vi "FGV RDB.vi"(9 "Raw data in":dbl[][](array[numeric]), 11 "Command":T1) -> (1 "Raw data out":dbl[][](array[numeric]), 3 "Size":i32)   [LabVIEW 2014]
uses:
  set-get-size.ctl
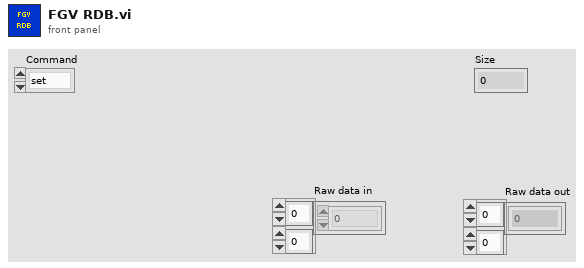
[diagram p1: front panel]
types:
  T1 = typedef "set-get-size.ctl" = enum16{"set", "get", "size"}
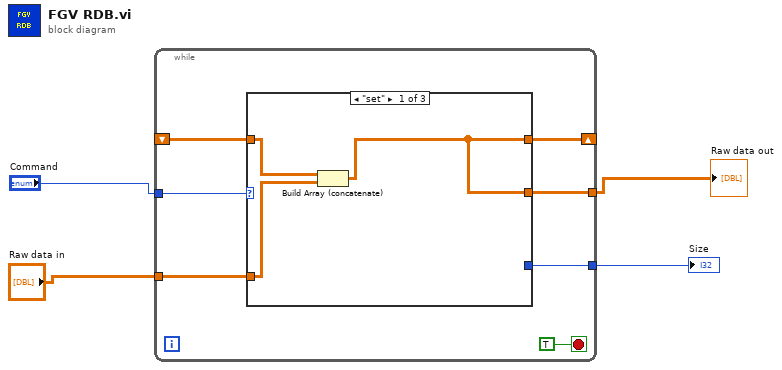
[diagram p0: block diagram]
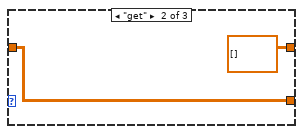
[diagram p2: hidden frame]
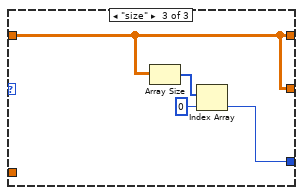
[diagram p3: hidden frame]
diagram:
  n1 = while {
    shift-right: [w8] -> _
    shift-left: _ -> [w9]
    tunnel: "Command" -> [w10]
    tunnel: "Raw data in" -> [w7]
    tunnel: [w6] -> w3
    tunnel: [w5] -> w1
    stop <- TRUE stop-if-true
    n2 = case shown="\"set\"" w10 {
      tunnel: w9 -> [w13 w16 w20]
      tunnel: [w12 dbl[][] [] w20] -> w8
      tunnel: w7 -> [w14 _ _]
      tunnel: [w12 w16 w20] -> w6
      tunnel: [_ _ w17] -> w5
      frame "set" {
        n3 = Build Array (concatenate)(w13, w14) -> (w12:dbl[][])
      }
      frame "get" {
      }
      frame "size" {
        n4 = Array Size(array=w20) -> (size(s)=w19:i32[])
        n5 = Index Array(array=w19, index=0) -> (element=w17:i32)
      }
    }
  }
  "Raw data out" <- w3
  "Size" <- w1
